vi "Read Text.vi"(6 "error in (no error)":errorcluster, 8 "timeout ms (5000)":i32=5000, 9 "Websocket Handler in":refnum<class "Websocket Handler.lvclass">) -> (0 "error out":errorcluster, 1 "String":string, 3 "Websocket Handler out":refnum<class "Websocket Handler.lvclass">)   [LabVIEW 2020, in "wamplv.lvlib" / "Websocket Handler.lvclass"]
uses:
  Websocket Handler.lvclass
  <vilib>/MediaMongrels Ltd/WebSockets/WebSockets/WebSocket Client/WebSocket Client.lvclass
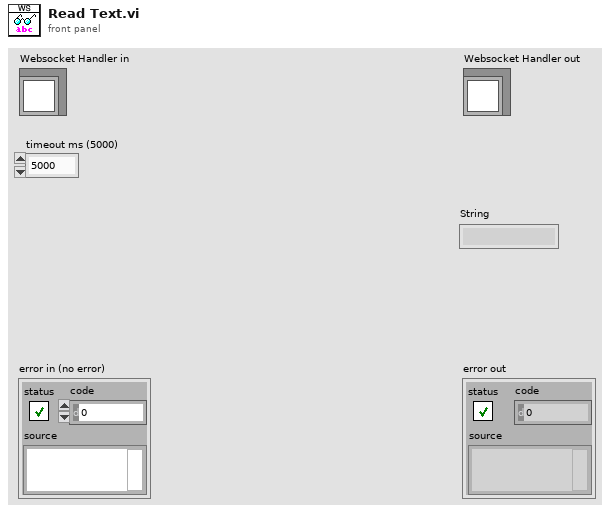
[diagram p1: front panel]
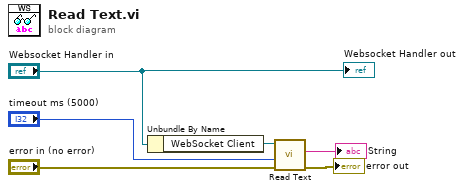
[diagram p0: block diagram]
diagram:
  n1 = Unbundle By Name("Websocket Handler in") -> ("WebSocket Client"=w2:refnum<class "WebSocket Client.lvclass">)
  n2 = call-dynamic "Read Text.vi"("error in (no error)"="error in (no error)", "timeout ms (5000)"="timeout ms (5000)", "WebSocket in"=w2) -> ("error out"=→"error out":errorcluster, "Data"=→"String":string)  [unwired: 6 in, 1 out]
  "Websocket Handler out" <- "Websocket Handler in"
